vi "Nattify - Ensure Leftmost BD Object Is Visible.vi"(0 "VI in":refnum<vi>, 1 "BD canvas margin":i16, 11 "error in":errorcluster) -> (15 "error out":errorcluster)   [LabVIEW 2020]
uses:
  <vilib>/Utility/miscctls.llb/LVPointTypeDef.ctl
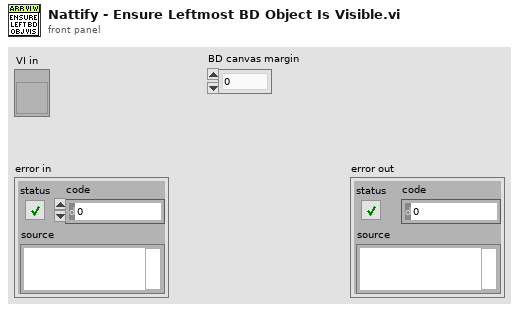
[diagram p1: front panel]
types:
  T1 = typedef "LVBoundsTypeDef.ctl" = cluster{"Width":u32, "Height":u32}
  T2 = typedef "LVRectTypeDef.ctl" = cluster{"Left":i16, "Top":i16, "Right":i16, "Bottom":i16}
  T3 = typedef "LVPointTypeDef.ctl" = cluster{"Horizontal":i16, "Vertical":i16}
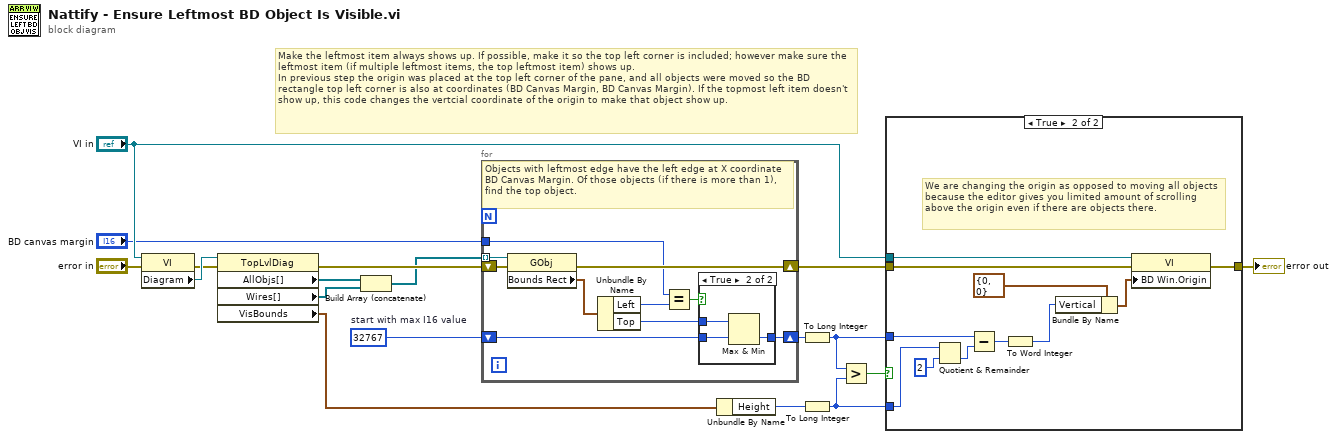
[diagram p0: block diagram]
diagram:
  w10 = i16 32767  # start with max I16 value
  # "Make the leftmost item always shows up. If possible, make it so the top left corner is included; however make sure the leftmost item (if multiple leftmost items, the top leftmost item) shows up.\nIn previous step the origin was placed at the top left corner of the pane, and all objects were moved so the BD rectangle top left corner is also at coordinates (BD Canvas Margin, BD Canvas Margin). If the topmost left item doesn't show up, this code changes the vertcial coordinate of the origin to make that object show up."
  n1 = property on="Property Node" class="VI"(reference="VI in", error in="error in") -> (error out=w17:errorcluster, "Diagram"=w18:refnum<vi>)  [unwired: 1 out]
  n2 = property on="Property Node" class="TopLvlDiag"(reference=w18, error in=w17) -> (error out=w4:errorcluster, "AllObjs[]"=w11:refnum<vi>[], "Wires[]"=w1:refnum<vi>[], "VisBounds"=w13:T1)  [unwired: 1 out]
  n3 = Build Array (concatenate)(w11, w1) -> (w2:refnum<vi>[])
  n4 = for {
    shift-right: [w26] -> w12
    shift-left: w4 -> [w28]
    shift-right: [w25] -> w6
    shift-left: w10 -> [w24]
    tunnel: w2 -> [w23] mode=indexing
    tunnel: "BD canvas margin" -> [w19]
    # "Objects with leftmost edge have the left edge at X coordinate BD Canvas Margin. Of those objects (if there is more than 1), find the top object."
    n5 = property on="Property Node" class="GObj"(reference=w23, error in=w28) -> (error out=w26:errorcluster, "Bounds Rect"=w27:T2)  [unwired: 1 out]
    n6 = Unbundle By Name(w27) -> ("Left"=w21:i16, "Top"=w22:i16)
    n7 = Equal?(x=w19, y=w21) -> (x = y?=w20:bool)
    n8 = case shown="True" w20 {
      tunnel: [w29 w32] -> w25
      tunnel: w24 -> [w29 w31]
      tunnel: w22 -> [_ w30]
      frame False {
      }
      frame True {
        n9 = Max & Min(x=w30, y=w31) -> (min(x,y)=w32:i16)  [unwired: 1 out]
      }
    }
  }
  n10 = Unbundle By Name(w13) -> ("Height"=w14:u32)
  n11 = To Long Integer(number=w6) -> (32bit integer=w3:i32)
  n12 = To Long Integer(number=w14) -> (32bit integer=w7:i32)
  n13 = Greater?(x=w3, y=w7) -> (0:w8:bool)
  n14 = case shown="True" w8 {
    tunnel: w12 -> [w33 w40]
    tunnel: [w33 w41] -> w9
    tunnel: "VI in" -> [_ w36]
    tunnel: w3 -> [_ w37]
    tunnel: w7 -> [_ w43]
    frame False {
    }
    frame True {
      # "We are changing the origin as opposed to moving all objects because the editor gives you limited amount of scrolling above the origin even if there are objects there."
      n15 = Quotient & Remainder(x=w43, y=2) -> (floor(x/y)=w42:i32)  [unwired: 1 out]
      n16 = Subtract(x=w37, y=w42) -> (x-y=w38:i32)
      n17 = To Word Integer(number=w38) -> (16bit integer=w34:i16)
      n18 = Bundle By Name(cluster=T3 {"Horizontal"=0, "Vertical"=0} ("Block Diagram Window:Origin"), "Vertical"=w34) -> (w35:T3)
      n19 = property on="Property Node" class="VI"(reference=w36, error in=w40, "BD Win.Origin"=w35) -> (error out=w41:errorcluster)  [unwired: 1 out]
    }
  }
  "error out" <- w9
